vi "peis.vi"(0 "IP adress":string="192.109.209.229", 1 "stop":bool, 2 "Channel":u8(ring) items=["1", "2", "3", "4", "5", "6", "7", "8", "9", "10", "11", "12", "13", "14", "15", "16"], 3 "SPEIS Parameters":T2={"Step_number"=0, "Initial_Voltage_step"=0.0, "vs_initial"=TRUE, "Final_Voltage_step"=1.0, "vs_final"=FALSE, "Duration_step"=1.0, "Record_every_dI"=0.1, "Record_every_dT"=0.1, "Initial_frequency"=100000.0, "sweep"=FALSE, "Final_frequency"=1.0, "Frequency_number"=51, "Amplitude_Voltage"=0.01, "Wait_for_steady"=2.0, "Average_N_times"=1, "Correction"=TRUE, "I_Range"=12, "Bandwidth"=5, "em"=1, "ce"=0} {"ce" items=["Standard", "CE to ground"]; "Initial_Voltage_step" min=-10 max=10 format="%.5f"; "Step_number" min=0 step=1; "I_Range" items=["1pA", "1nA", "10nA", "100nA", "1µA", "10µA", "100µA", "1mA", "10mA", "100mA", "1A", "Booster", "Auto"]; "Wait_for_steady" min=0 format="%.2f"; "Record_every_dT" min=0 format="%.2e"; "Record_every_dI" min=0 format="%.2e"; "Duration_step" min=0 format="%.5f"; "Final_Voltage_step" min=-10 max=10 format="%.5f"; "Bandwidth" items=["1"=1, "2"=2, "3"=3, "4"=4, "5"=5, "6"=6, "7"=7, "8"=8, "9"=9]; "Average_N_times" min=1 max=1000 step=1; "Amplitude_Voltage" min=0.0005 max=0.5 format="%.2e"; "Final_frequency" min=1e-05 max=1000000 format="%.2e"; "Frequency_number" min=1 max=10000; "Initial_frequency" min=1e-05 max=1000000 format="%.2e"}, 4 "Exit":bool, 5 "Start":bool, 8 "Draw":T1(ring)) -> (6 "XY Graph":cluster{"Data p1":sgl[], "Data p1":dbl[]}[](graph), 7 "Number of points":i32=52)   [LabVIEW 2012]
doc: "The Staircase Potentio Electrochemical Impedance Spectroscopy (SPEIS) technique is designed to perform successive impedance measurements (on a whole frequency range) during a potential sweep. \nThis technique consists in a staircase potential sweep (potential limits and number of steps defined by the user). An impedance measurement (with an adjustable number of frequencies) is performed on each potential step.\n\nIn general, in this VI, the first thing to do is to start by establishing the connection with the instrument defined by its IP adress, then load the firmware in the channel selected, get the information on the plugged channels, load protocol on a channel, start/stop the protocol, retreive data and draw the graph.\nThis technique is applied just for channels with impedance capabilities (Zboard)."
uses:
  base_xml.llb/Type Descriptor Enumeration__ogtk.ctl
panel:
  out "Data p0":sgl[][](array[numeric])=[[0.100008, 0.099745475, 1.9343544e-05], [0.200016, 0.09966919, 1.936642e-05], [0.300024, 0.10005063, 1.9374045e-05], [0.400032, 0.10005063, 1.9358795e-05], [0.50004, 0.09997434, 1.9358795e-05], [0.600048, 0.09982177, 1.938167e-05], [0.700056, 0.099516615, 1.9358795e-05], [0.800064, 0.099898055, 1.9374045e-05], [0.90007204, 0.099516615, 1.936642e-05]]
  out "Data p1":sgl[][](array[numeric])=[[99999.99, 0.009897927, 1.5485124e-05, -0.23932889, 0.09957624, 2.0601647e-05, 0.0, 0.017584162, 1.5528842e-05, -0.13801742, -0.10928005, -2.0601661e-05, 0.0, 1.89, 7.0], [79789.055, 0.009909321, 1.4999416e-05, -0.28277892, 0.09956935, 2.0610883e-05, 0.0, 0.017358849, 1.5026583e-05, -0.16497254, -0.10927754, -2.0610896e-05, 0.0, 2.319, 7.0], [63671.867, 0.00993305, 1.4371862e-05, -0.3338619, 0.099571265, 2.0617736e-05, 0.0, 0.01701651, 1.4388475e-05, -0.19887781, -0.10927467, -2.0617748e-05, 0.0, 2.748, 7.0], [50804.684, 0.009895762, 1.349999e-05, -0.38682938, 0.099595726, 2.0621628e-05, 0.0, 0.016509676, 1.3509973e-05, -0.23511207, -0.10929042, -2.0621641e-05, 0.0, 3.177, 7.0], [40539.06, 0.009924297, 1.2531375e-05, -0.43154812, 0.09956674, 2.0623062e-05, 0.0, 0.01605967, 1.2537333e-05, -0.27001935, -0.1092824, -2.0623074e-05, 0.0, 3.606, 7.0], [32343.752, 0.009929493, 1.1422184e-05, -0.4605673, 0.099575475, 2.0627644e-05, 0.0, 0.015497766, 1.1425662e-05, -0.29694676, -0.10927959, -2.0627656e-05, 0.0, 4.035, 7.0], [25812.496, 0.009931898, 1.0332502e-05, -0.47349262, 0.09957423, 2.0616248e-05, 0.0, 0.014982226, 1.0334525e-05, -0.31350675, -0.10928383, -2.0616259e-05, 0.0, 4.4639997, 7.0], [20593.748, 0.009683827, 9.104932e-06, -0.46709442, 0.09957324, 2.0613099e-05, 0.0, 0.014134236, 9.106069e-06, -0.3174526, -0.10928545, -2.0613114e-05, 0.0, 4.75, 7.0], [16429.69, 0.00984061, 8.381006e-06, -0.4425385, 0.0995779, 2.0614962e-05, 0.0, 0.013980997, 8.381673e-06, -0.30736777, -0.10928426, -2.0614974e-05, 0.0, 5.036, 7.0], [13109.373, 0.009880392, 7.759602e-06, -0.4042132, 0.09956233, 2.0629059e-05, 0.0, 0.013766184, 7.759997e-06, -0.28469434, -0.10927877, -2.0629072e-05, 0.0, 5.322, 7.0], [10460.936, 0.009915135, 7.290463e-06, -0.35881066, 0.099576354, 2.062228e-05, 0.0, 0.013552605, 7.2907023e-06, -0.25464892, -0.10927802, -2.0622294e-05, 0.0, 5.608, 7.0], [8351.5625, 0.009958473, 6.968417e-06, -0.30687237, 0.09957134, 2.0619169e-05, 0.0, 0.013452288, 6.968562e-06, -0.21966934, -0.10928822, -2.0619183e-05, 0.0, 5.894, 7.0], [6660.1553, 0.009773157, 6.585265e-06, -0.26302314, 0.09957721, 2.0628519e-05, 0.0, 0.013077308, 6.5853465e-06, -0.18975565, -0.109301746, -2.0628531e-05, 0.0, 6.0620003, 7.0], [5313.953, 0.009875495, 6.4977903e-06, -0.21722555, 0.09959636, 2.061105e-05, 0.0, 0.013129692, 6.497844e-06, -0.15612268, -0.10930546, -2.0611064e-05, 0.0, 6.269, 7.0], [4241.786, 0.009916322, 6.4091464e-06, -0.17841792, 0.09959986, 2.0643229e-05, 0.0, 0.013149473, 6.4091746e-06, -0.12683374, -0.109303646, -2.0643243e-05, 0.0, 6.4830003, 7.0], [3385.4163, 0.009962957, 6.371731e-06, -0.15283132, 0.09959816, 2.0641255e-05, 0.0, 0.013166811, 6.371748e-06, -0.11219756, -0.10930573, -2.0641268e-05, 0.0, 6.697, 7.0], [2699.3184, 0.009985389, 6.3324687e-06, -0.12883663, 0.099599674, 2.0642745e-05, 0.0, 0.013169419, 6.3324833e-06, -0.09362733, -0.10931173, -2.0642758e-05, 0.0, 6.9110003, 7.0], [2153.4448, 0.009996085, 6.3133293e-06, -0.11305499, 0.09959159, 2.0643656e-05, 0.0, 0.013185124, 6.313335e-06, -0.08275235, -0.109307505, -2.064367e-05, 0.0, 7.125, 7.0], [1717.748, 0.010014333, 6.2567524e-06, -0.10080016, 0.09959457, 2.0655203e-05, 0.0, 0.013182044, 6.256763e-06, -0.07431483, -0.10931141, -2.0655216e-05, 0.0, 7.34, 7.0], [1372.1951, 0.010016238, 6.2877625e-06, -0.09321749, 0.09959682, 2.064688e-05, 0.0, 0.013175669, 6.2877634e-06, -0.06877315, -0.10931128, -2.0646892e-05, 0.0, 7.5550003, 7.0], [1096.7545, 0.010012516, 6.286433e-06, -0.08541584, 0.09960139, 2.0640491e-05, 0.0, 0.013178928, 6.2864306e-06, -0.062073976, -0.10930484, -2.0640506e-05, 0.0, 7.77, 7.0], [871.93097, 0.010010969, 6.268487e-06, -0.08781743, 0.09959833, 2.0634905e-05, 0.0, 0.013172707, 6.2684835e-06, -0.06440747, -0.109307244, -2.0634918e-05, 0.0, 7.987, 7.0], [696.1138, 0.01003125, 6.2508416e-06, -0.093888, 0.09959319, 2.0650714e-05, 0.0, 0.013164024, 6.2508466e-06, -0.069969416, -0.10931639, -2.0650728e-05, 0.0, 8.203, 7.0], [555.8894, 0.010025321, 6.2520185e-06, -0.10746312, 0.099596396, 2.063822e-05, 0.0, 0.01315077, 6.2520166e-06, -0.08037281, -0.109306626, -2.0638234e-05, 0.0, 8.42, 7.0], [443.43906, 0.010033136, 6.209101e-06, -0.12175393, 0.0995993, 2.0631758e-05, 0.0, 0.01312816, 6.2091035e-06, -0.091670275, -0.109299496, -2.063177e-05, 0.0, 8.639, 7.0], [353.75473, 0.01003465, 6.1840165e-06, -0.14335668, 0.09959073, 2.0645593e-05, 0.0, 0.013097799, 6.1840187e-06, -0.10758209, -0.10931424, -2.0645608e-05, 0.0, 8.859, 7.0], [281.8943, 0.010030967, 6.109471e-06, -0.17281115, 0.09959446, 2.0650212e-05, 0.0, 0.013065848, 6.109473e-06, -0.129511, -0.10930905, -2.0650225e-05, 0.0, 9.0789995, 7.0], [225.3606, 0.010023677, 6.0119432e-06, -0.20512176, 0.09959748, 2.064375e-05, 0.0, 0.013001974, 6.0119396e-06, -0.15545309, -0.1093129, -2.0643763e-05, 0.0, 9.301, 7.0], [180.28844, 0.010028235, 5.913567e-06, -0.25207758, 0.0995884, 2.0643136e-05, 0.0, 0.012923154, 5.913563e-06, -0.19031943, -0.1093126, -2.0643149e-05, 0.0, 9.526, 7.0], [143.75787, 0.010025335, 5.723294e-06, -0.2980666, 0.09959362, 2.0638052e-05, 0.0, 0.012791262, 5.7232987e-06, -0.22673774, -0.109312676, -2.0638066e-05, 0.0, 9.755, 7.0], [114.59661, 0.0100282775, 5.478785e-06, -0.36026663, 0.09959826, 2.0642558e-05, 0.0, 0.012615283, 5.4787893e-06, -0.27884817, -0.109307505, -2.0642572e-05, 0.0, 9.987, 7.0], [91.552734, 0.010020258, 5.1631105e-06, -0.41180015, 0.09958356, 2.0632298e-05, 0.0, 0.012400166, 5.1631077e-06, -0.32256132, -0.10930771, -2.0632311e-05, 0.0, 10.219, 7.0], [72.87778, 0.010045694, 4.7920767e-06, -0.47027957, 0.0995903, 1.9318108e-05, 0.0, 0.012195916, 4.7920753e-06, -0.37585485, -0.10930665, -1.931812e-05, 0.0, 10.735, 6.0], [58.30223, 0.010017018, 4.3459513e-06, -0.5196618, 0.09958969, 1.931711e-05, 0.0, 0.011869716, 4.345951e-06, -0.41790736, -0.109305374, -1.9317124e-05, 0.0, 10.989, 6.0], [46.50297, 0.010043655, 3.8964367e-06, -0.5461425, 0.09958527, 1.9321726e-05, 0.0, 0.011661541, 3.8964395e-06, -0.45622373, -0.10929812, -1.9321737e-05, 0.0, 11.24, 6.0], [36.95101, 0.0100237075, 3.4589034e-06, -0.55786407, 0.09959118, 1.9322812e-05, 0.0, 0.011445447, 3.4589052e-06, -0.47548974, -0.1093029, -1.9322824e-05, 0.0, 11.498, 6.0], [29.592804, 0.010024518, 3.0782626e-06, -0.5442606, 0.099590674, 1.9320825e-05, 0.0, 0.011281099, 3.0782635e-06, -0.4723431, -0.10930497, -1.9320838e-05, 0.0, 11.782001, 6.0], [23.588463, 0.010025413, 2.7635026e-06, -0.50970626, 0.09959939, 1.931987e-05, 0.0, 0.011168829, 2.7635024e-06, -0.45203626, -0.10930516, -1.9319881e-05, 0.0, 12.092, 6.0], [18.780045, 0.010028319, 2.5114025e-06, -0.46162716, 0.0995976, 1.9318664e-05, 0.0, 0.01109292, 2.5114036e-06, -0.4128492, -0.109315775, -1.9318675e-05, 0.0, 12.425, 6.0], [15.024037, 0.010029642, 2.331001e-06, -0.4064955, 0.099582985, 1.9321948e-05, 0.0, 0.01104459, 2.3310024e-06, -0.36793888, -0.10930361, -1.9321958e-05, 0.0, 12.772, 6.0], [11.982363, 0.010013976, 2.1986236e-06, -0.3445742, 0.0995901, 1.9318428e-05, 0.0, 0.01101896, 2.198625e-06, -0.31417423, -0.10929007, -1.931844e-05, 0.0, 13.119, 6.0], [9.574144, 0.010021789, 2.1110484e-06, -0.29042864, 0.09959056, 1.931938e-05, 0.0, 0.011009957, 2.1110482e-06, -0.26570365, -0.10930588, -1.9319392e-05, 0.0, 13.55, 6.0], [7.6293964, 0.010015764, 2.047544e-06, -0.2358973, 0.09959619, 1.9324216e-05, 0.0, 0.010986972, 2.0475438e-06, -0.21676749, -0.10930043, -1.9324229e-05, 0.0, 14.088, 6.0], [6.084501, 0.010008753, 2.0095065e-06, -0.19609833, 0.09960107, 1.9321422e-05, 0.0, 0.010978085, 2.0095063e-06, -0.17923641, -0.10930903, -1.9321435e-05, 0.0, 14.758, 6.0], [4.858519, 0.0100127505, 1.9834858e-06, -0.15383446, 0.099605374, 1.9325236e-05, 0.0, 0.01099137, 1.983485e-06, -0.14275539, -0.10930968, -1.9325249e-05, 0.0, 15.594, 6.0], [3.8752477, 0.010018873, 1.964741e-06, -0.12660927, 0.09960577, 1.9319072e-05, 0.0, 0.01098087, 1.9647398e-06, -0.11773729, -0.10930894, -1.9319084e-05, 0.0, 16.639, 6.0], [3.1001983, 0.01002199, 1.954336e-06, -0.101673305, 0.09960291, 1.9318823e-05, 0.0, 0.010977447, 1.9543347e-06, -0.09406805, -0.10931086, -1.9318833e-05, 0.0, 17.943, 6.0], [2.4660668, 0.010017678, 1.9471984e-06, -0.08063111, 0.09960053, 1.9318097e-05, 0.0, 0.010982101, 1.9471975e-06, -0.07494378, -0.10931104, -1.9318108e-05, 0.0, 19.579, 6.0], [1.9649143, 0.01001538, 1.9460967e-06, -0.064157724, 0.09960199, 1.9316354e-05, 0.0, 0.010980325, 1.946096e-06, -0.06017399, -0.1093061, -1.9316365e-05, 0.0, 21.627, 6.0], [1.5725644, 0.010012327, 1.941652e-06, -0.051375534, 0.09960348, 1.9317453e-05, 0.0, 0.010977772, 1.9416514e-06, -0.04843211, -0.10930792, -1.9317464e-05, 0.0, 24.183, 6.0], [1.2520034, 0.010019626, 1.939335e-06, -0.041469768, 0.09961237, 1.9318904e-05, 0.0, 0.010981496, 1.9393347e-06, -0.038478374, -0.109313786, -1.9318915e-05, 0.0, 27.391, 6.0], [1.0016024, 0.010014649, 1.938777e-06, -0.033258826, 0.09960662, 1.931856e-05, 0.0, 0.010977961, 1.9387764e-06, -0.031450033, -0.109310396, -1.9318572e-05, 0.0, 31.398, 6.0]]
  out "Exit 2":bool=TRUE
  # "Instructions:\nBefore running the VI you must type a valid IP adress that corresponds to the instrument.Then press the Run button to execute this VI.\nWhile this VI is running, choose the available channel, enter the SPEIS parameters or keep the default\n values, then press the start button to begin the experience. \nChoose the waveform to draw : Nyquist, modZ, theta...\nPress the stop button to end experience and the exit button to stop the VI execution."
  # "Set E (V)  vs. previous"
  # "Before EIS  stay for ts (s)"
  # "and record every dI (A)"
  # "or every dt (s)"
  # "Start EIS from  Fi (Hz)"
  # "sweep linear/logarithmic"
  # "to Ff (Hz)"
  # "for Nf frequencies"
  # "with the amplitude (V)"
  # "wait for Pw"
  # "average Na times"
  # "drift correction"
  # "with I Range"
  # "and bandwidth"
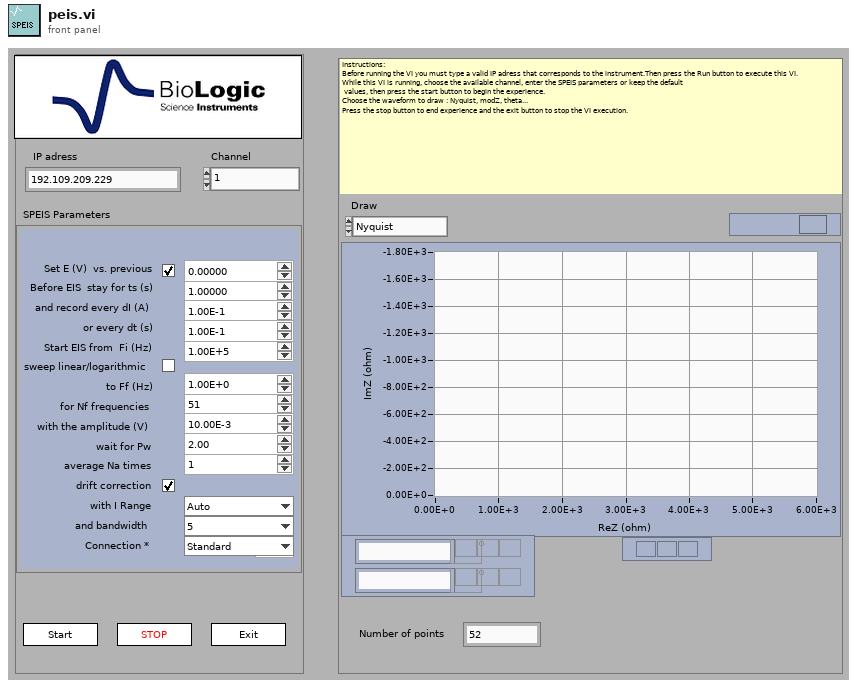
[diagram p1: front panel]
types:
  T1 = enum16{"Nyquist", "modZ", "theta", "modE", "modI", "Edc", "Idc", "E range", "I range", "f(t)"}
  T2 = cluster{"Step_number":i32, "Initial_Voltage_step":sgl, "vs_initial":bool, "Final_Voltage_step":sgl, "vs_final":bool, "Duration_step":sgl, "Record_every_dI":sgl, "Record_every_dT":sgl, "Initial_frequency":sgl, "sweep":bool, "Final_frequency":sgl, "Frequency_number":i32, "Amplitude_Voltage":sgl, "Wait_for_steady":sgl, "Average_N_times":i32, "Correction":bool, "I_Range":u16, "Bandwidth":u16, "em":u16, "ce":u16}
  T3 = typedef "Type Descriptor Enumeration__ogtk.ctl" = enum8{"<Null>", "I8", "I16", "I32", "I64", "U8", "U16", "U32", "U64", "SGL", "DBL", "EXT", "CSG", "CDB", "CXT", "0x0F", "0x10", "0x11", "0x12", "0x13", "0x14", "Enum U8", "Enum U16", "Enum U32", "Enum U64", "SGL PQ", "DBL PQ", "EXT PQ", "CSG PQ", "CDB PQ", "CXT PQ", "0x1F", "0x20", "Boolean", "0x22", "0x23", "0x24", "0x25", "0x26", "0x27", "0x28", "0x29", "0x2A", "0x2B", "0x2C", "0x2D", "0x2E", "0x2F", "String", "0x31", "Path", "Pict", "0x34", "0x35", "0x36", "DAQ", "0x38", "0x39", "0x3A", "0x3B", "0x3C", "0x3D", "0x3E", "0x3F", "Array", "0x41", "0x42", "0x43", "0x44", "0x45", "0x46", "0x47", "0x48", "0x49", "0x4A", "0x4B", "0x4C", "0x4D", "0x4E", "0x4F", "Cluster", "0x51", "0x52", "Variant", "Waveform", "0x55", "0x56", "0x57", "0x58", "0x59", "0x5A", "0x5B", "0x5C", "0x5D", "0x5E", "0x5F", "0x60", "0x61", "0x62", "0x63", "0x64", "0x65", "0x66", "0x67", "0x68", "0x69", "0x6A", "0x6B", "0x6C", "0x6D", "0x6E", "0x6F", "Refnum"}
  T4 = cluster{"Data Type":T3, "Format String":string}[]
  T5 = cluster{"Channel":i32, "BoardVersion":i32, "BoardSerialCode":i32, "FirmwareCode":i32, "FirmwareVersion":i32, "XilinxVersion":i32, "AmpCode":i32, "NbAmp":i32, "LcBoard":i32, "Zboard":i32, "MuxBoard":i32, "GPRAboard":i32, "MemSize":i32, "MemFilled":i32, "state":i32, "MaxIRange":i32, "MinIRange":i32, "MaxBandwidth":i32, "NbOfTechniques":i32}
  T6 = cluster{"Label":string, "type":i32, "valeur":u32, "index":i32}[]
  T7 = cluster{"IRQskipped":i32, "NbRaws":i32, "NbCols":i32, "Technique Index":i32, "TechniqueID":i32, "PrcessIndex":i32, "loop":i32, "StartTime":dbl, "MuxPad":i32}
  T8 = cluster{"State":i32, "MemFilled":i32, "TimeBase":sgl, " Ewe":sgl, " EweRangeMin":sgl, " EweRangeMax":sgl, "Ece":sgl, "EceRangeMin":sgl, "EceRangeMax":sgl, "Eoverflow":i32, "I":sgl, "IRange":i32, "Ioverflow":i32, "ElapsedTime":sgl, "Freq":sgl, "Rcomp":sgl, "Saturation":sgl, "OptErr":i32, "OptPos":i32}
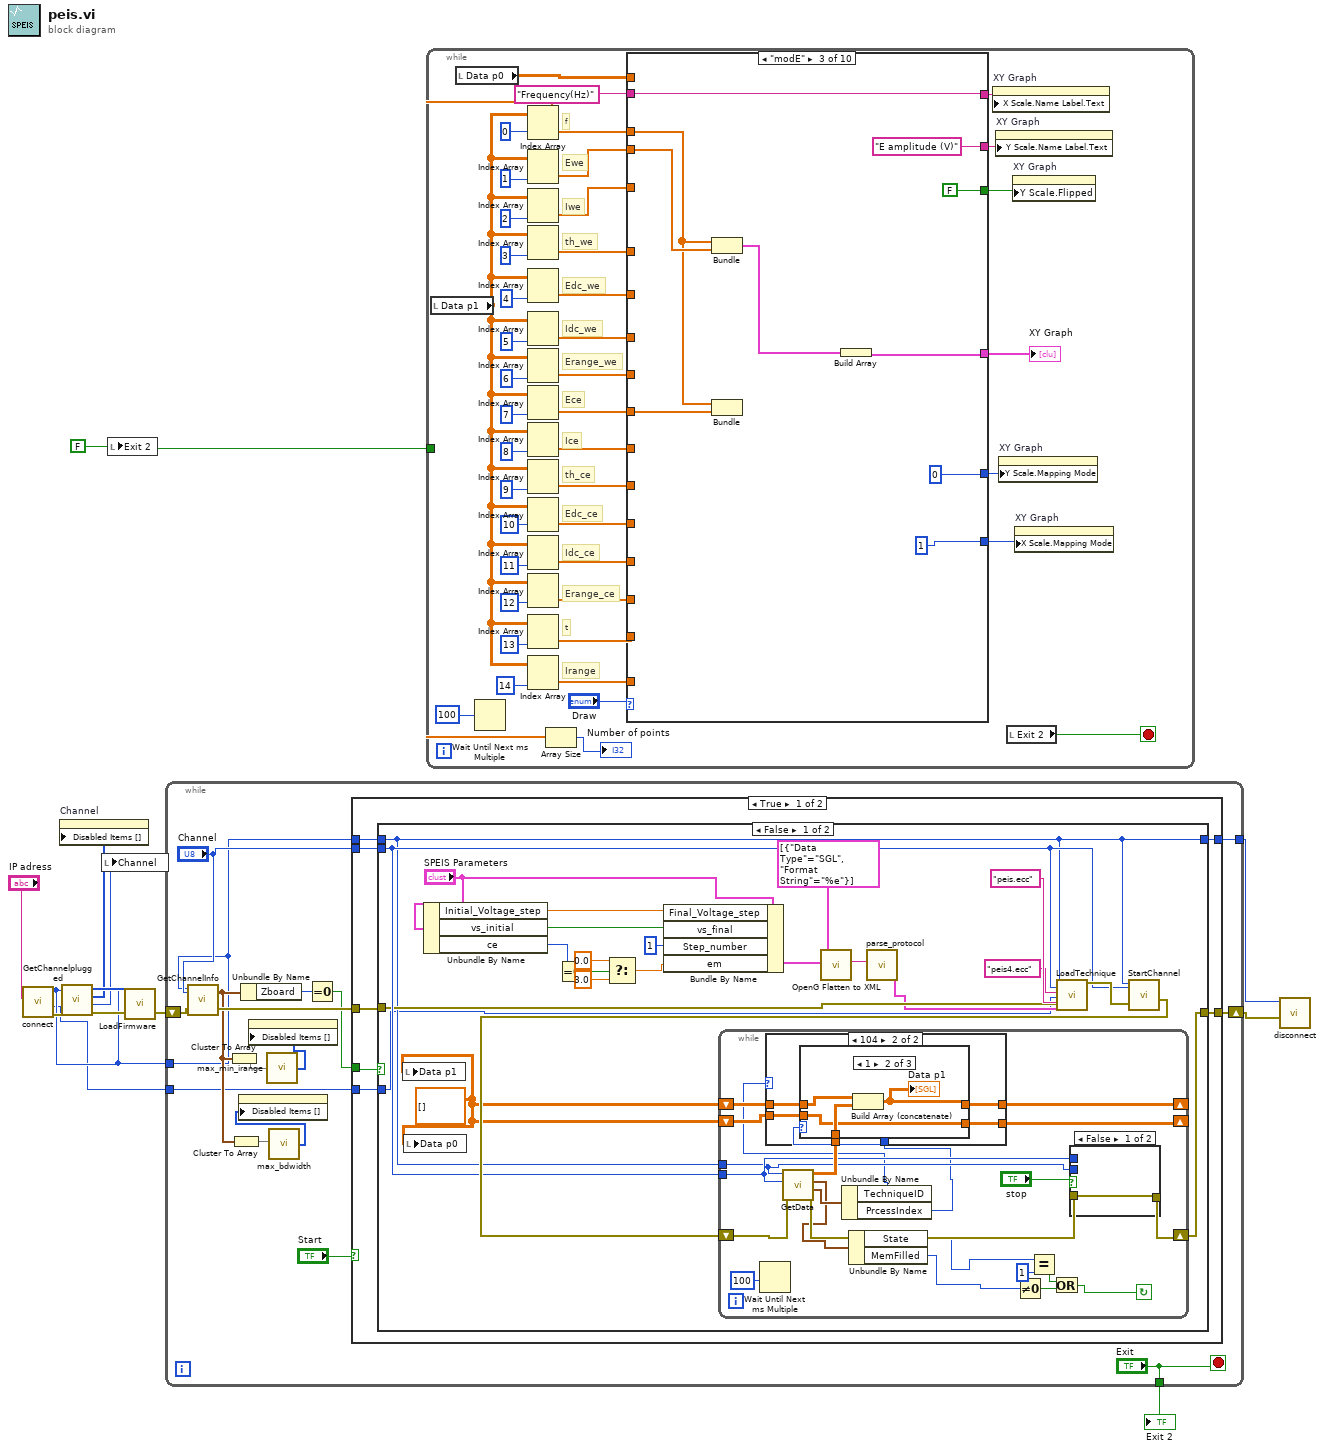
[diagram p0: block diagram]
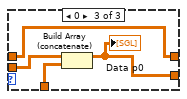
[diagram p4: hidden frame]
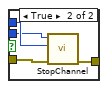
[diagram p5: hidden frame]
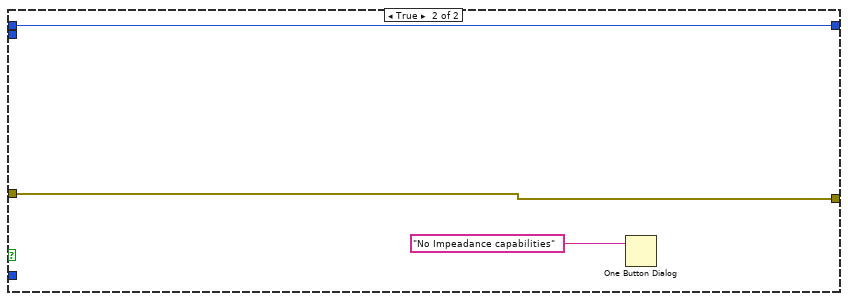
[diagram p6: hidden frame]
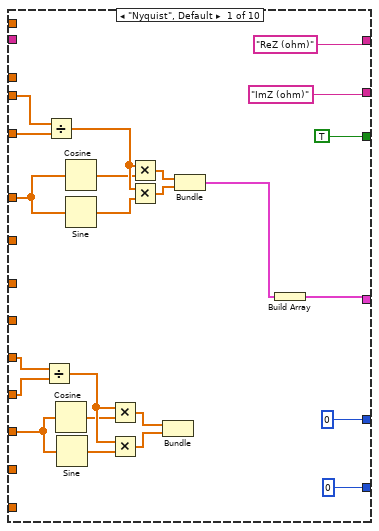
[diagram p8: hidden frame]
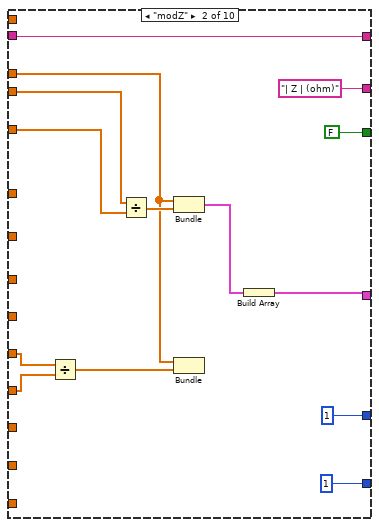
[diagram p9: hidden frame]
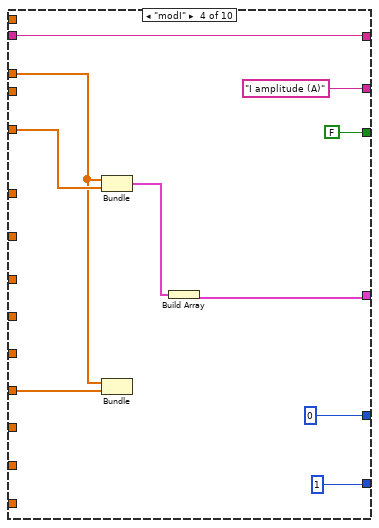
[diagram p10: hidden frame]
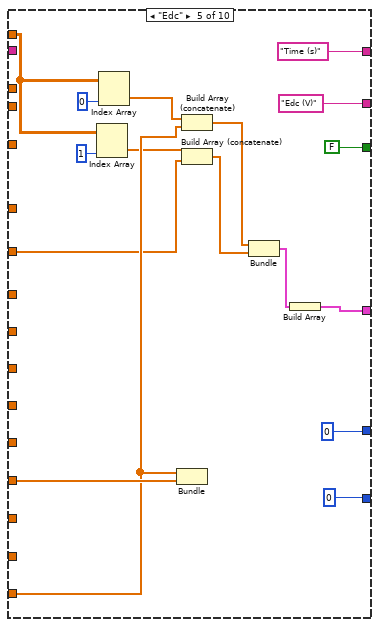
[diagram p11: hidden frame]
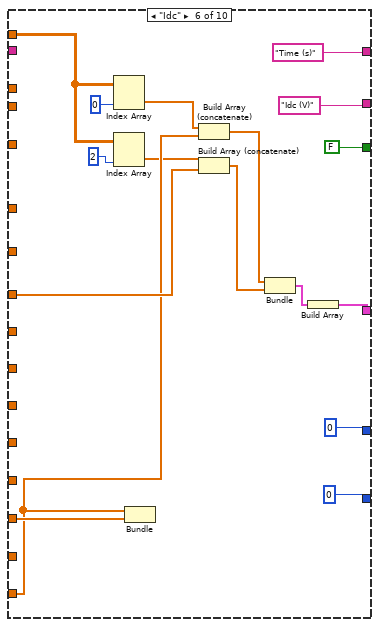
[diagram p12: hidden frame]
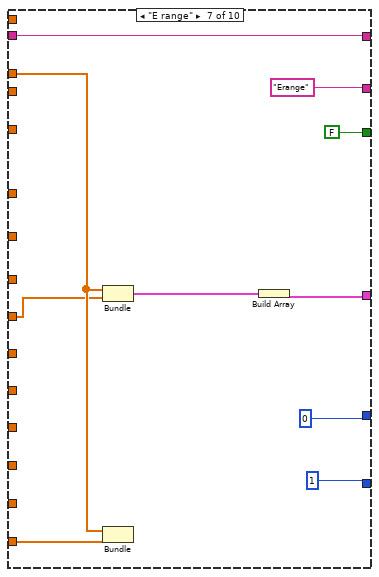
[diagram p13: hidden frame]
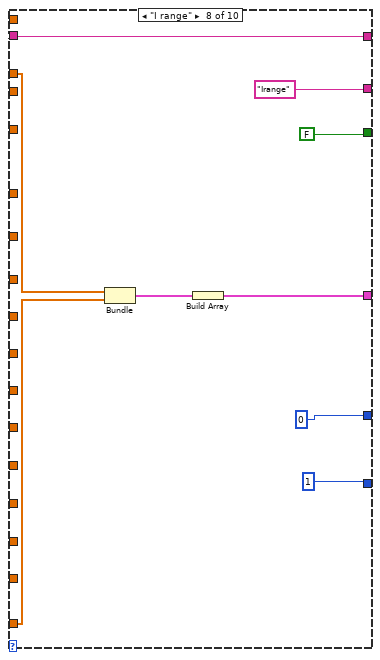
[diagram p14: hidden frame]
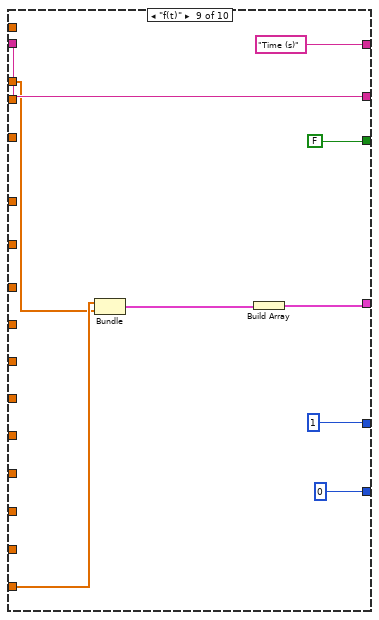
[diagram p15: hidden frame]
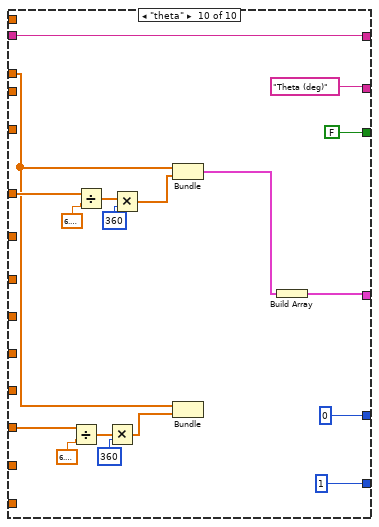
[diagram p16: hidden frame]
diagram:
  w6 = FALSE
  n1 = call "connect.vi"("IP"="IP adress") -> ("error out"=w12:errorcluster, "Device Code"=w1:i32, "ID"=w3:i32)  [unwired: 7 in, 1 out]
  n2 = call "GetChannelplugged.vi"("error in (no error)"=w12, "ID"=w3) -> ("error out"=w10:errorcluster, "First channel"=w8:i32, "Disabled channels"=w7:i32[], "Plugged channels"=w11:i32[])  [unwired: 6 in]
  n3 = property on="Channel" class="Ring (strict)"("Disabled Items []"=w7) -> ()  [unwired: 2 in, 2 out]
  n4 = local write "Channel"(w8) -> ()
  n5 = local write "Exit 2"(w6) -> ()
  n6 = call "LoadFirmware.vi"("error in (no error)"=w10, "Channels"=w11, "ID"=w3) -> ("error out"=w4:errorcluster)  [unwired: 7 in, 1 out]
  n7 = while {
    shift-right: [w28] -> w13
    shift-left: w4 -> [w23]
    tunnel: ["Exit"] -> w5
    tunnel: w3 -> [w16]
    tunnel: [w15] -> w2
    tunnel: w1 -> [w14]
    stop <- "Exit" stop-if-true
    n8 = call "GetChannelInfo.vi"("error in (no error)"=w23, "Channel"="Channel", "ID"=w16) -> ("error out"=w22:errorcluster, "Channel information"=w20:T5)  [unwired: 7 in]
    n9 = Cluster To Array(cluster=w20) -> (array=w26:i32[])
    n10 = Cluster To Array(cluster=w20) -> (array=w19:i32[])
    n11 = Unbundle By Name(w20) -> ("Zboard"=w25:i32)
    n12 = call "max_min_irange.vi"("resources"=w26) -> ("disabled ranges"=w17:i32[])
    n13 = property on="I_Range" class="Ring (strict)"("Disabled Items []"=w17) -> ()  [unwired: 2 in, 2 out]
    n14 = call "max_bdwidth.vi"("resources"=w19) -> ("disabled ranges"=w18:i32[])
    n15 = property on="Bandwidth" class="Ring (strict)"("Disabled Items []"=w18) -> ()  [unwired: 2 in, 2 out]
    n16 = Equal To 0?(x=w25) -> (x = 0?=w21:bool)
    n17 = case shown="True" "Start" {
      tunnel: "Channel" -> [w35 _]
      tunnel: [w36 w109] -> w28
      tunnel: w22 -> [w34 w109]
      tunnel: w21 -> [w33 _]
      tunnel: w16 -> [w32 w108]
      tunnel: [w31 w108] -> w15
      tunnel: w14 -> [w30 _]
      frame True {
        n18 = case shown="False" w33 {
          tunnel: [w56 w106] -> w36
          tunnel: w35 -> [w55 _]
          tunnel: w34 -> [w54 w106]
          tunnel: w32 -> [w49 w105]
          tunnel: [w49 w105] -> w31
          tunnel: w30 -> [w48 _]
          frame False {
            w53 = sgl[][] [] ("Data")
            n19 = local write "Data p1"(w53) -> ()
            n20 = local write "Data p0"(w53) -> ()
            n21 = Unbundle By Name("SPEIS Parameters") -> ("Initial_Voltage_step"=w44:sgl, "vs_initial"=w43:bool, "ce"=w38:u16)
            n22 = Equal To 0?(x=w38) -> (x = 0?=w39:bool)
            n23 = Select(t=0.0, s=w39, f=3.0) -> (s? t:f=w37:dbl)
            n24 = Bundle By Name(cluster="SPEIS Parameters", "Final_Voltage_step"=w44, "vs_final"=w43, "Step_number"=1, "em"=w37) -> (w45:T2)
            n25 = call "OpenG Flatten to XML.vi"("Type Formats (default)"=T4 [{"Data Type"=enum."SGL", "Format String"="%e"}] ("Type Formats"), "LabVIEW Data"=w45) -> ("XML String"=w52:string)  [unwired: 8 in, 1 out]
            n26 = call "parse_protocol.vi"("XML String In"=w52) -> ("Params Values"=w51:T6)  [unwired: 8 in]
            n27 = call "LoadTechnique.vi"("ID"=w49, "Selected Channel"=w55, "FName4"="peis4.ecc" ("FName"), "Device Code"=w48, "FName"="peis.ecc", "Protocol Parameters"=w51, "error in (no error)"=w54) -> ("error out"=w58:errorcluster)  [unwired: 12 in]
            n28 = call "StartChannel.vi"("error in (no error)"=w58, "Channel"=w55, "ID"=w49) -> ("error out"=w57:errorcluster)  [unwired: 8 in]
            n29 = while {
              shift-right: [w76] -> w56
              shift-left: w57 -> [w78]
              tunnel: w55 -> [w67]
              shift-right: [w71] -> _
              shift-left: w53 -> [w72]
              shift-right: [w70] -> _
              shift-left: w53 -> [w69]
              tunnel: w49 -> [w66]
              stop <- w74 continue-if-true
              n30 = Wait Until Next ms Multiple(millisecond multiple=u32 100) -> ()  [unwired: 1 out]
              n31 = call "GetData.vi"("error in (no error)"=w78, "Channel"=w67, "ID"=w66) -> ("error out"=w75:errorcluster, "Data information"=w65:T7, "Current values"=w61:T8, "Data"=w73:dbl[][])  [unwired: 5 in]
              n32 = Unbundle By Name(w65) -> ("TechniqueID"=w64:i32, "PrcessIndex"=w60:i32)
              n33 = case shown="104" w64 {
                tunnel: w73 -> [_ w89]
                tunnel: w72 -> [w83 w88]
                tunnel: [w83 w87] -> w71
                tunnel: [w82 w86] -> w70
                tunnel: w69 -> [w82 w85]
                tunnel: w60 -> [_ w84]
                frame 0, Default {
                }
                frame 104 {
                  n34 = case shown="1" w84 {
                    tunnel: w89 -> [_ w95 w99]
                    tunnel: w88 -> [w91 w94 w96]
                    tunnel: [w91 w93 w96] -> w87
                    tunnel: [w90 w92 w98] -> w86
                    tunnel: w85 -> [w90 w92 w97]
                    frame 2, Default {
                    }
                    frame 1 {
                      n35 = Build Array (concatenate)(w94, w95) -> (w93:dbl[][])
                      "Data p1" <- w93
                    }
                    frame 0 {
                      n36 = Build Array (concatenate)(w97, w99) -> (w98:dbl[][])
                      "Data p0" <- w98
                    }
                  }
                }
              }
              n37 = Unbundle By Name(w61) -> ("State"=w63:i32, "MemFilled"=w62:i32)
              n38 = Not Equal To 0?(x=w62) -> (x != 0?=w79:bool)
              n39 = Equal?(x=w63, y=1) -> (x = y?=w80:bool)
              n40 = Or(x=w80, y=w79) -> (x .or. y?=w74:bool)
              n41 = case shown="False" "stop" {
                tunnel: [w100 w104] -> w76
                tunnel: w75 -> [w100 w103]
                tunnel: w67 -> [_ w102]
                tunnel: w66 -> [_ w101]
                frame False {
                }
                frame True {
                  n42 = call "StopChannel.vi"("error in (no error)"=w103, "Channel"=w102, "ID"=w101) -> ("error out"=w104:errorcluster)  [unwired: 8 in]
                }
              }
            }
          }
          frame True {
            n43 = One Button Dialog(message="No Impeadance capabilities" ("error source (\" \")")) -> ()  [unwired: 1 in, 1 out]
          }
        }
      }
      frame False {
      }
    }
  }
  "Exit 2" <- w5
  n44 = while {
    tunnel: w6 -> [_]
    stop <- w141 stop-if-true
    # "Erange_ce"
    # "Idc_ce"
    # "Edc_ce"
    # "th_ce"
    # "Ice"
    # "Ece"
    # "t"
    # "Irange"
    # "Erange_we"
    # "Idc_we"
    # "Edc_we"
    # "th_we"
    # "Iwe"
    # "Ewe"
    # "f"
    n45 = local read "Data p1"() -> (w126:sgl[][])
    n46 = local read "Data p0"() -> (w113:sgl[][])
    n47 = Wait Until Next ms Multiple(millisecond multiple=u32 100) -> ()  [unwired: 1 out]
    n48 = Index Array(array=w126, index (col)=0 ("Index")) -> (element=w112:sgl[])  [unwired: 1 in]
    n49 = Index Array(array=w126, index (col)=1 ("Index")) -> (element=w127:sgl[])  [unwired: 1 in]
    n50 = Index Array(array=w126, index (col)=2 ("Index")) -> (element=w131:sgl[])  [unwired: 1 in]
    n51 = Index Array(array=w126, index (col)=3 ("Index")) -> (element=w146:sgl[])  [unwired: 1 in]
    n52 = Index Array(array=w126, index (col)=4 ("disabled index (col)")) -> (element=w140:sgl[])  [unwired: 1 in]
    n53 = Index Array(array=w126, index (col)=5 ("disabled index (col)")) -> (element=w137:sgl[])  [unwired: 1 in]
    n54 = Index Array(array=w126, index (col)=6 ("index (row)")) -> (element=w128:sgl[])  [unwired: 1 in]
    n55 = Index Array(array=w126, index (col)=7) -> (element=w119:sgl[])  [unwired: 1 in]
    n56 = Index Array(array=w126, index (col)=8) -> (element=w118:sgl[])  [unwired: 1 in]
    n57 = Index Array(array=w126, index (col)=9) -> (element=w117:sgl[])  [unwired: 1 in]
    n58 = Index Array(array=w126, index (col)=10) -> (element=w116:sgl[])  [unwired: 1 in]
    n59 = Index Array(array=w126, index (col)=11) -> (element=w115:sgl[])  [unwired: 1 in]
    n60 = Index Array(array=w126, index (col)=12) -> (element=w114:sgl[])  [unwired: 1 in]
    n61 = Index Array(array=w126, index (col)=13 ("disabled index (col)")) -> (element=w129:sgl[])  [unwired: 1 in]
    n62 = Index Array(array=w126, index (col)=14 ("disabled index (col)")) -> (element=w130:sgl[])  [unwired: 1 in]
    n63 = Array Size(array=w112) -> (size(s)=→"Number of points":i32)
    n64 = case shown="\"modE\"" "Draw" {
      tunnel: w112 -> [_ w178 w192 w203 _ _ w248 w256 w265 w274]
      tunnel: w127 -> [w175 w189 w199 _ _ _ _ _ _ _]
      tunnel: w131 -> [w174 w182 _ w209 _ _ _ _ _ _]
      tunnel: ["ImZ (ohm)" ("Y Scale.Name Label.Text") "| Z | (ohm)" ("Y Scale.Name Label.Text") "E amplitude (V)" ("Y Scale.Name Label.Text") "I amplitude (A)" ("Y Scale.Name Label.Text") "Edc (V)" ("Y Scale.Name Label.Text") "Idc (V)" ("Y Scale.Name Label.Text") "Erange" ("Y Scale.Name Label.Text") "Irange" ("Y Scale.Name Label.Text") w270 "Theta (deg)" ("Y Scale.Name Label.Text")] -> w148
      tunnel: w146 -> [w173 _ _ _ _ _ _ _ _ w283]
      tunnel: ["ReZ (ohm)" ("Y Scale.Name Label.Text") w186 w197 w207 "Time (s)" ("Y Scale.Name Label.Text") "Time (s)" ("Y Scale.Name Label.Text") w253 w262 "Time (s)" ("Y Scale.Name Label.Text") w289] -> w145
      tunnel: "Frequency(Hz)" ("Y Scale.Name Label.Text") -> [_ w186 w197 w207 _ _ w253 w262 w270 w289]
      tunnel: [TRUE ("Y Scale.Flipped") FALSE ("Y Scale.Flipped") FALSE ("Y Scale.Flipped") FALSE ("Y Scale.Flipped") FALSE ("Y Scale.Flipped") FALSE ("Y Scale.Flipped") FALSE ("Y Scale.Flipped") FALSE FALSE FALSE ("Y Scale.Flipped")] -> w143
      tunnel: [u8 0 ("X Scale.Mapping Mode") u8 1 ("X Scale.Mapping Mode") u8 1 ("X Scale.Mapping Mode") u8 1 ("X Scale.Mapping Mode") 0 0 1 1 0 u8 1 ("X Scale.Mapping Mode")] -> w142
      tunnel: w140 -> [_ _ _ _ w210 _ _ _ _ _]
      tunnel: w137 -> [_ _ _ _ _ w231 _ _ _ _]
      tunnel: w128 -> [_ _ _ _ _ _ w244 _ _ _]
      tunnel: w130 -> [_ _ _ _ _ _ _ w257 _ _]
      tunnel: w129 -> [_ _ _ _ w212 w230 _ _ w266 _]
      tunnel: [0 1 u8 0 ("X Scale.Mapping Mode") u8 0 ("X Scale.Mapping Mode") 0 0 0 0 1 0 ("X Scale.Mapping Mode")] -> w133
      tunnel: w119 -> [w164 w180 w193 _ _ _ _ _ _ _]
      tunnel: w118 -> [w163 w179 _ w202 _ _ _ _ _ _]
      tunnel: w117 -> [w162 _ _ _ _ _ _ _ _ w275]
      tunnel: w116 -> [_ _ _ _ w222 _ _ _ _ _]
      tunnel: w115 -> [_ _ _ _ _ w239 _ _ _ _]
      tunnel: w114 -> [_ _ _ _ _ _ w245 _ _ _]
      tunnel: [w156 w176 w190 w200 w221 w237 w246 w254 w263 w272] -> w110
      tunnel: w113 -> [_ _ _ _ w215 w233 _ _ _ _]
      frame "Nyquist", Default {
        n65 = Divide(x=w164, y=w163) -> (x/y=w158:sgl[])
        n66 = Divide(x=w175, y=w174) -> (x/y=w160:sgl[])
        n67 = Cosine(x=w162) -> (cos(x)=w157:sgl[])
        n68 = Sine(x=w162) -> (sin(x)=w165:sgl[])
        n69 = Cosine(x=w173) -> (cos(x)=w159:sgl[])
        n70 = Sine(x=w173) -> (sin(x)=w155:sgl[])
        n71 = Multiply(x=w158, y=w157) -> (x*y=w167:sgl[])
        n72 = Multiply(x=w158, y=w165) -> (x*y=w166:sgl[])
        n73 = Multiply(x=w160, y=w159) -> (x*y=w154:sgl[])
        n74 = Multiply(x=w160, y=w155) -> (x*y=w153:sgl[])
        n75 = Bundle(w167, w166) -> ()  [unwired: 1 in, 1 out]
        n76 = Bundle(w154, w153) -> (w161:cluster{sgl[], sgl[]})  [unwired: 1 in]
        n77 = Build Array(w161) -> (w156:cluster{sgl[], sgl[]}[])
      }
      frame "modZ" {
        n78 = Divide(x=w180, y=w179) -> (x/y=w181:sgl[])
        n79 = Divide(x=w189, y=w182) -> (x/y=w188:sgl[])
        n80 = Bundle("Data p1"=w178, w188) -> (w177:cluster{"Data p1":sgl[], sgl[]})  [unwired: 1 in]
        n81 = Bundle("Data p1"=w178, w181) -> ()  [unwired: 1 in, 1 out]
        n82 = Build Array(w177) -> (w176:cluster{"Data p1":sgl[], sgl[]}[])
      }
      frame "modE" {
        n83 = Bundle("Data p1"=w192, "Data p1"=w199) -> (w191:cluster{"Data p1":sgl[], "Data p1":sgl[]})  [unwired: 1 in]
        n84 = Bundle("Data p1"=w192, "Data p1"=w193) -> ()  [unwired: 1 in, 1 out]
        n85 = Build Array(w191) -> (w190:cluster{"Data p1":sgl[], "Data p1":sgl[]}[])
      }
      frame "modI" {
        n86 = Bundle("Data p1"=w203, "Data p1"=w209) -> (w201:cluster{"Data p1":sgl[], "Data p1":sgl[]})  [unwired: 1 in]
        n87 = Bundle("Data p1"=w203, "Data p1"=w202) -> ()  [unwired: 1 in, 1 out]
        n88 = Build Array(w201) -> (w200:cluster{"Data p1":sgl[], "Data p1":sgl[]}[])
      }
      frame "Edc" {
        n89 = Index Array(array=w215, index (col)=1 ("Index")) -> (element=w211:sgl[])  [unwired: 1 in]
        n90 = Index Array(array=w215, index (col)=0 ("Index")) -> (element=w213:sgl[])  [unwired: 1 in]
        n91 = Bundle("Data p1"=w212, "Data p1"=w222) -> ()  [unwired: 1 in, 1 out]
        n92 = Build Array (concatenate)(w213, w212) -> (w218:sgl[])
        n93 = Build Array (concatenate)(w211, w210) -> (w217:sgl[])
        n94 = Bundle(w218, w217) -> (w214:cluster{sgl[], sgl[]})  [unwired: 1 in]
        n95 = Build Array(w214) -> (w221:cluster{sgl[], sgl[]}[])
      }
      frame "Idc" {
        n96 = Index Array(array=w233, index (col)=0 ("Index")) -> (element=w232:sgl[])  [unwired: 1 in]
        n97 = Index Array(array=w233, index (col)=2 ("Index")) -> (element=w229:sgl[])  [unwired: 1 in]
        n98 = Bundle("Data p1"=w230, "Data p1"=w239) -> ()  [unwired: 1 in, 1 out]
        n99 = Build Array (concatenate)(w232, w230) -> (w228:sgl[])
        n100 = Build Array (concatenate)(w229, w231) -> (w227:sgl[])
        n101 = Bundle(w228, w227) -> (w238:cluster{sgl[], sgl[]})  [unwired: 1 in]
        n102 = Build Array(w238) -> (w237:cluster{sgl[], sgl[]}[])
      }
      frame "E range" {
        n103 = Bundle("Data p1"=w248, "Data p1"=w244) -> (w247:cluster{"Data p1":sgl[], "Data p1":sgl[]})  [unwired: 1 in]
        n104 = Bundle("Data p1"=w248, "Data p1"=w245) -> ()  [unwired: 1 in, 1 out]
        n105 = Build Array(w247) -> (w246:cluster{"Data p1":sgl[], "Data p1":sgl[]}[])
      }
      frame "I range" {
        n106 = Bundle("Data p1"=w256, "Data p1"=w257) -> (w255:cluster{"Data p1":sgl[], "Data p1":sgl[]})  [unwired: 1 in]
        n107 = Build Array(w255) -> (w254:cluster{"Data p1":sgl[], "Data p1":sgl[]}[])
      }
      frame "f(t)" {
        n108 = Bundle("Data p1"=w266, "Data p1"=w265) -> (w264:cluster{"Data p1":sgl[], "Data p1":sgl[]})  [unwired: 1 in]
        n109 = Build Array(w264) -> (w263:cluster{"Data p1":sgl[], "Data p1":sgl[]}[])
      }
      frame "theta" {
        n110 = Divide(x=w275, y=6.283185307179586) -> (x/y=w277:dbl[])
        n111 = Divide(x=w283, y=6.283185307179586) -> (x/y=w286:dbl[])
        n112 = Multiply(x=w277, y=360) -> (x*y=w279:dbl[])
        n113 = Multiply(x=w286, y=360) -> (x*y=w282:dbl[])
        n114 = Bundle("Data p1"=w274, w282) -> (w273:cluster{"Data p1":sgl[], dbl[]})  [unwired: 1 in]
        n115 = Bundle("Data p1"=w274, w279) -> ()  [unwired: 1 in, 1 out]
        n116 = Build Array(w273) -> (w272:cluster{"Data p1":sgl[], dbl[]}[])
      }
    }
    "XY Graph" <- w110
    n117 = property on="XY Graph" class="XYGraph (strict)"("X Scale.Name Label.Text"=w145) -> ()  [unwired: 2 in, 2 out]
    n118 = property on="XY Graph" class="XYGraph (strict)"("Y Scale.Name Label.Text"=w148) -> ()  [unwired: 2 in, 2 out]
    n119 = property on="XY Graph" class="XYGraph (strict)"("Y Scale.Mapping Mode"=w133) -> ()  [unwired: 2 in, 2 out]
    n120 = local read "Exit 2"() -> (w141:bool)
    n121 = property on="XY Graph" class="XYGraph (strict)"("Y Scale.Flipped"=w143) -> ()  [unwired: 2 in, 2 out]
    n122 = property on="XY Graph" class="XYGraph (strict)"("X Scale.Mapping Mode"=w142) -> ()  [unwired: 2 in, 2 out]
  }
  n123 = call "disconnect.vi"("error in (no error)"=w13, "ID"=w2) -> ()  [unwired: 9 in, 1 out]
